vi "Main On Load Action VI.vi"(8 "error in (no error)":errorcluster, 11 "Device Item Ref in":T1 format="%.0x") -> (0 "error out":errorcluster, 3 "Device Item Ref out":T1 format="%.0x")   [LabVIEW 2015, in "Engine Simulation Toolkit System Explorer.lvlib"]
uses:
  Engine Simulation Toolkit System Explorer.lvlib
  <vilib>/NI Veristand/Custom Device API/Custom Device Item Ref.ctl
  NationalInstruments.VeriStand.SystemDefinitionAPI
  Shared/Constants and GUIDs.vi
  Shared/Properties.vi
  <vilib>/NI Veristand/Custom Device API/Get Item Property (String).vi
  <vilib>/NI Veristand/Custom Device API/Set Item Property (String).vi
  <vilib>/NI Veristand/Custom Device API/Get Item Property (Dependent File).vi
  <vilib>/NI Veristand/Custom Device API/Set Item Property (Dependent File).vi
  <vilib>/NI Veristand/Custom Device API/Custom Device API.lvlib
  Shared/Engine Simulation Toolkit Shared.lvlib
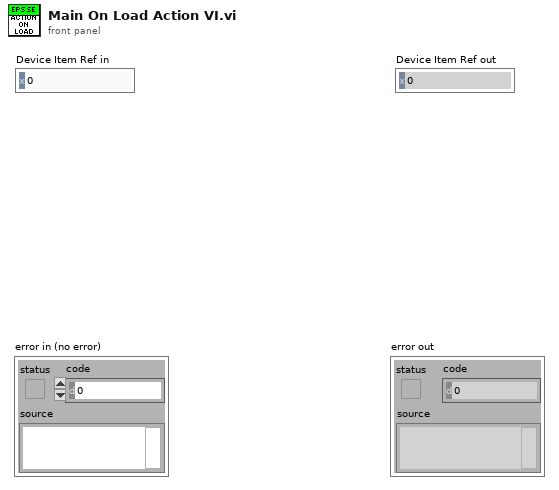
[diagram p1: front panel]
types:
  T1 = typedef "Custom Device API.lvlib/Custom Device Item Ref.ctl" = u64
  T2 = typedef "Custom Device API.lvlib/Dependent File Optional Info.ctl" = cluster{"Version":string, "RTDestination":path, "ForceDownload":bool, "SupportedTarget":string, "MD5":string}
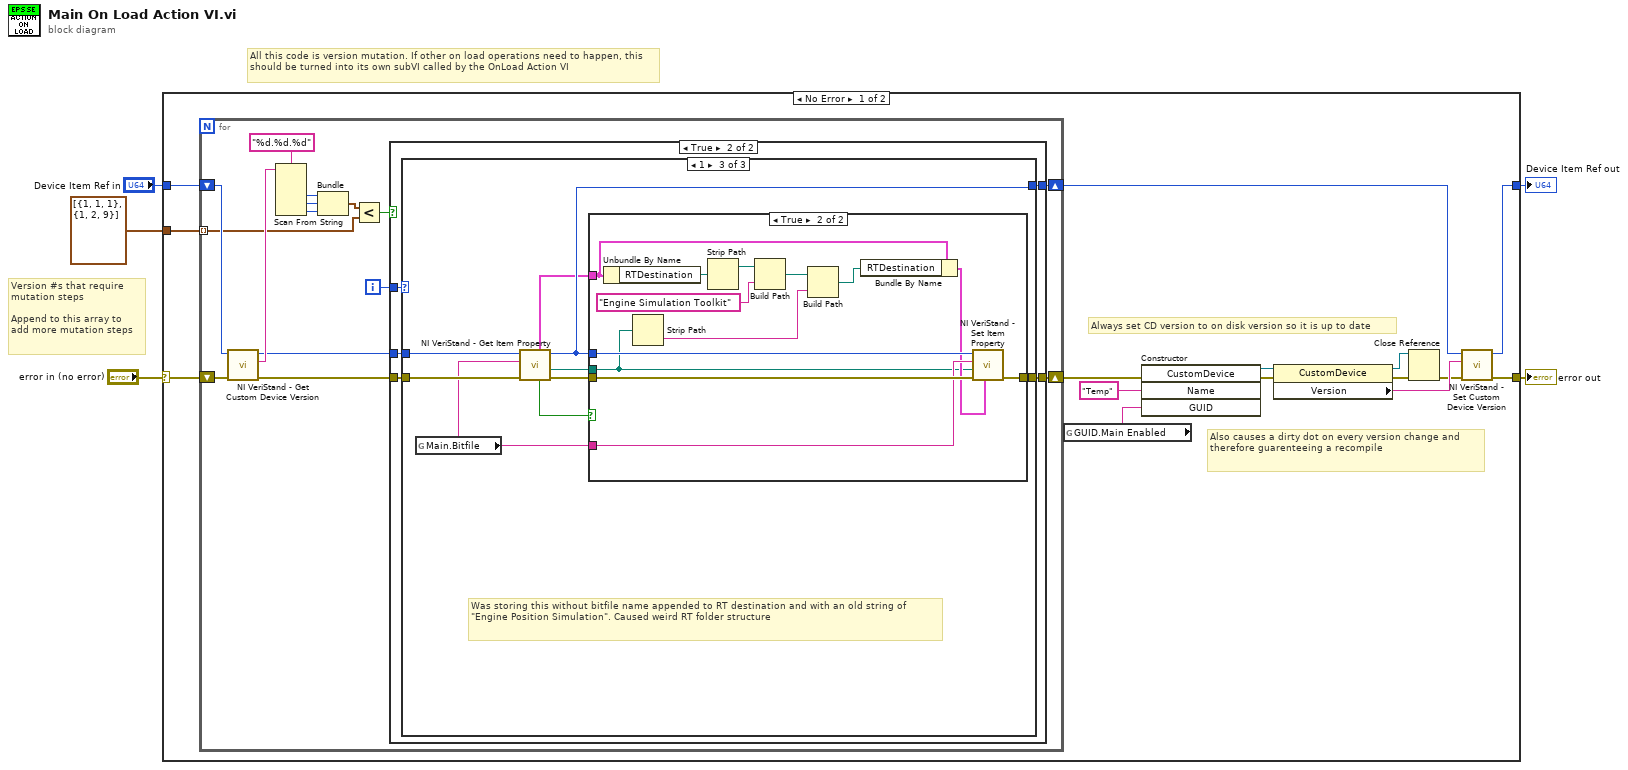
[diagram p0: block diagram]
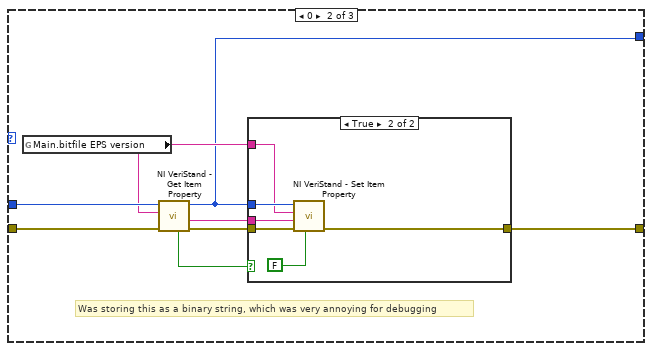
[diagram p4: hidden frame]
diagram:
  # "All this code is version mutation. If other on load operations need to happen, this should be turned into its own subVI called by the OnLoad Action VI"
  # "Version #s that require\nmutation steps\n\nAppend to this array to\nadd more mutation steps"
  n1 = case shown="No Error" "error in (no error)" {
    selector: "error in (no error)" -> [w19 w84]
    tunnel: [w9 w84] -> w4
    tunnel: "Device Item Ref in" -> [w18 w83]
    tunnel: [w7 w83] -> w2
    tunnel: cluster{i32, i32, i32}[] [{1, 1, 1}, {1, 2, 9}] -> [w20 _]
    frame No Error {
      # "Also causes a dirty dot on every version change and therefore guarenteeing a recompile"
      # "Always set CD version to on disk version so it is up to date"
      n2 = for {
        tunnel: w20 -> [w22] mode=indexing
        shift-right: [w26] -> w10
        shift-left: w19 -> [w31]
        shift-right: [w24] -> w8
        shift-left: w18 -> [w30]
        i -> [w23]
        n3 = call <vilib>:"NI VeriStand - Get Custom Device Version.vi"("error in (no error)"=w31, "Device Ref in"=w30) -> ("error out"=w27:errorcluster, "Value"=w29:string, "Device Ref out"=w25:T1)  [unwired: 7 in]
        n4 = Scan From String(format string="%d.%d.%d", input string=w29) -> (output 1=w33:i32, output 2=w34:i32, output 3=w21:i32)  [unwired: 5 in, 3 out]
        n5 = Bundle(w33, w34, w21) -> (w35:cluster{i32, i32, i32})  [unwired: 1 in]
        n6 = Less?(x=w35, y=w22) -> (x < y?=w28:bool)
        n7 = case shown="True" w28 {
          tunnel: w27 -> [w37 w42]
          tunnel: [w37 w41] -> w26
          tunnel: w25 -> [w36 w38]
          tunnel: [w36 w39] -> w24
          tunnel: w23 -> [_ w40]
          frame False {
          }
          frame True {
            n8 = case shown="1" w40 {
              tunnel: w42 -> [w44 w51 w67]
              tunnel: [w44 w46 w62] -> w41
              tunnel: [w43 w45 w61] -> w39
              tunnel: w38 -> [w43 w52 w68]
              frame Default {
              }
              frame 0 {
                # "Was storing this as a binary string, which was very annoying for debugging"
                n9 = global read "Properties.vi" "Main.bitfile EPS version"() -> (w48:string)
                n10 = call-poly <vilib>:"NI VeriStand - Get Item Property.vi"("error in (no error)"=w51, "Property Name"=w48, "Item Ref in"=w52) -> ("error out"=w49:errorcluster, "Value"=w47:string, "Item Ref out"=w45:T1, "Found?"=w50:bool)  [unwired: 5 in]
                n11 = case shown="True" w50 {
                  tunnel: w45 -> [_ w59]
                  tunnel: w49 -> [w53 w58]
                  tunnel: w48 -> [_ w57]
                  tunnel: w47 -> [_ w56]
                  tunnel: [w53 w54] -> w46
                  frame False {
                  }
                  frame True {
                    n12 = call-poly <vilib>:"NI VeriStand - Set Item Property.vi"("Binary String (T)"=FALSE, "error in (no error)"=w58, "Value"=w56, "Property Name"=w57, "Item Ref in"=w59) -> ("error out"=w54:errorcluster)  [unwired: 4 in, 2 out]
                  }
                }
              }
              frame 1 {
                # "Was storing this without bitfile name appended to RT destination and with an old string of \"Engine Position Simulation\". Caused weird RT folder structure"
                n13 = global read "Properties.vi" "Main.Bitfile"() -> (w64:string)
                n14 = call-poly <vilib>:"NI VeriStand - Get Item Property.vi"("error in (no error)"=w67, "Property Name"=w64, "Item Ref in"=w68) -> ("error out"=w65:errorcluster, "Path"=w63:path, "Item Ref out"=w61:T1, "Found"=w66:bool, "OptionalInfo"=w60:T2)  [unwired: 4 in]
                n15 = case shown="True" w66 {
                  tunnel: w61 -> [_ w82]
                  tunnel: w65 -> [w69 w81]
                  tunnel: w64 -> [_ w80]
                  tunnel: w63 -> [_ w75]
                  tunnel: [w69 w79] -> w62
                  tunnel: w60 -> [_ w78]
                  frame False {
                  }
                  frame True {
                    n16 = Unbundle By Name(w78) -> ("RTDestination"=w74:path)
                    n17 = Strip Path(path=w75) -> (name=w76:string)  [unwired: 1 out]
                    n18 = Strip Path(path=w74) -> (stripped path=w73:path)  [unwired: 1 out]
                    n19 = Build Path(base path=w73, name or relative path="Engine Simulation Toolkit") -> (appended path=w72:path)
                    n20 = Build Path(base path=w72, name or relative path=w76) -> (appended path=w70:path)
                    n21 = Bundle By Name(cluster=w78, "RTDestination"=w70) -> (w77:T2)
                    n22 = call-poly <vilib>:"NI VeriStand - Set Item Property.vi"("OptionalInfo"=w77, "error in (no error)"=w81, "Path"=w75, "Property Name"=w80, "Item Ref in"=w82) -> ("error out"=w79:errorcluster)  [unwired: 4 in, 2 out]
                  }
                }
              }
            }
          }
        }
      }
      n23 = global read "Constants and GUIDs.vi" "GUID.Main Enabled"() -> (w6:string)
      n24 = constructor class="CustomDevice"(error in=w10, "Name"="Temp", "GUID"=w6) -> (reference out=w16:refnum<k24>, error out=w15:errorcluster)  [unwired: 2 in, 3 out]
      n25 = property class="CustomDevice"(reference=w16, error in=w15) -> (reference out=w13:refnum<k24>, error out=w14:errorcluster, "Version"=w12:string)
      n26 = Close Reference(reference=w13, error in (no error)=w14) -> (error out=w11:errorcluster)
      n27 = call <vilib>:"NI VeriStand - Set Custom Device Version.vi"("error in (no error)"=w11, "Value"=w12, "Device Ref in"=w8) -> ("error out"=w9:errorcluster, "Device Ref out"=w7:T1)  [unwired: 7 in]
    }
    frame Error {
    }
  }
  "error out" <- w4
  "Device Item Ref out" <- w2
